vi "_Validate Source Parameters.vi"(11 "Expts":string[][](array[string])=[["0", "MRM", "Positive", "234", "7199", "22", "5000", "20", "2", "70", "ESI1 5001"], ["1", "MRM", "Positive", "0", "4988", "22", "5000", "0", "2", "70", "APCI2 3.1"], ["2", "MRM", "Negative", "678", "9085", "22", "5000", "20", "2", "70", "ESI1 -4001"], ["3", "MRM", "Negative", "0", "7199", "22", "5000", "0", "2", "70", "APCI2 -3.2"]]) -> (1 "Error":string, 2 "SourceProperties":T2[](array[typedef])=[{"Source Type"=2, "IsPole1"=TRUE, "IsAPCI"=FALSE, "IsPositive"=TRUE, "CD"=0.0, "ES1"=5001.0, "ES2"=0.0, "NextCD"=0.0, "NextES1"=0.0, "NextES2"=0.0, "PolSwitching"=FALSE, "StartTime"=0.0, "StopTime"=7199.0, "DelayTime"=20.0, "Cycles"=0, "PauseTime"=0.0, "ExptDuration"=0.0}, {"Source Type"=1, "IsPole1"=FALSE, "IsAPCI"=TRUE, "IsPositive"=TRUE, "CD"=3.1, "ES1"=0.0, "ES2"=0.0, "NextCD"=0.0, "NextES1"=0.0, "NextES2"=0.0, "PolSwitching"=FALSE, "StartTime"=0.0, "StopTime"=7199.0, "DelayTime"=0.0, "Cycles"=0, "PauseTime"=0.0, "ExptDuration"=0.0}, {"Source Type"=2, "IsPole1"=TRUE, "IsAPCI"=FALSE, "IsPositive"=FALSE, "CD"=0.0, "ES1"=-4001.0, "ES2"=0.0, "NextCD"=0.0, "NextES1"=0.0, "NextES2"=0.0, "PolSwitching"=FALSE, "StartTime"=0.0, "StopTime"=7199.0, "DelayTime"=20.0, "Cycles"=0, "PauseTime"=0.0, "ExptDuration"=0.0}, {"Source Type"=1, "IsPole1"=FALSE, "IsAPCI"=TRUE, "IsPositive"=FALSE, "CD"=-3.2, "ES1"=0.0, "ES2"=0.0, "NextCD"=0.0, "NextES1"=0.0, "NextES2"=0.0, "PolSwitching"=FALSE, "StartTime"=0.0, "StopTime"=7199.0, "DelayTime"=0.0, "Cycles"=0, "PauseTime"=0.0, "ExptDuration"=0.0}] {"Source Type" items=["APCI 1", "APCI 2", "ESI 1", "ESI 2"]}, 3 "Valid":bool)   [LabVIEW 2012]
uses:
  _Source Properties.ctl
  _XML Source Type.ctl
panel:
  out "PeriodList":T1(array[cluster])
  out "Time array":dbl[](array[numeric])
  # "Num             Type            Polarity        StartTime      StopTime        Cycles       PauseTime    DelayTime      ExptDur      DwellTime   Comment"
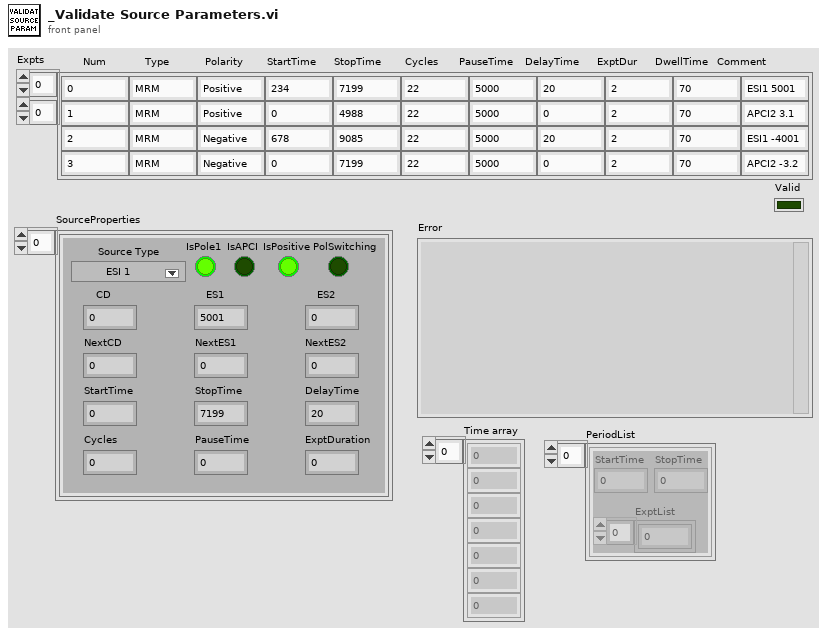
[diagram p1: front panel]
types:
  T1 = cluster{"StartTime":dbl, "StopTime":dbl, "ExptList":i32[]}[]
  T2 = typedef "_Source Properties.ctl" = cluster{"Source Type":T3, "IsPole1":bool, "IsAPCI":bool, "IsPositive":bool, "CD":dbl, "ES1":dbl, "ES2":dbl, "NextCD":dbl, "NextES1":dbl, "NextES2":dbl, "PolSwitching":bool, "StartTime":dbl, "StopTime":dbl, "DelayTime":dbl, "Cycles":i32, "PauseTime":dbl, "ExptDuration":dbl}
  T3 = typedef "_XML Source Type.ctl" = u16
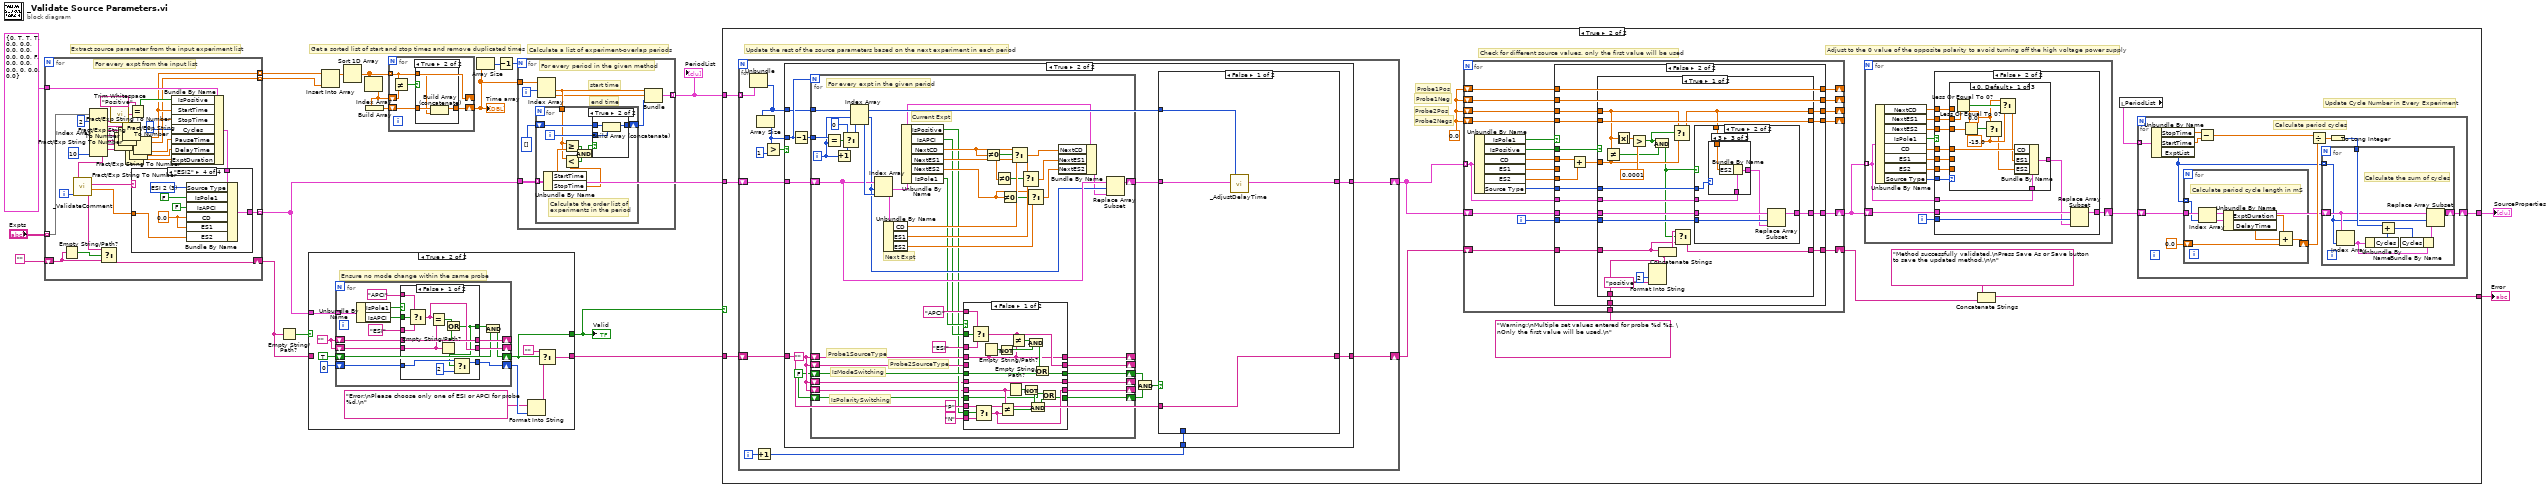
[diagram p0: block diagram]
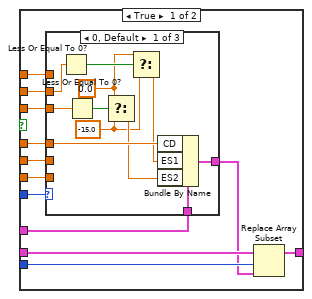
[diagram p3: hidden frame]
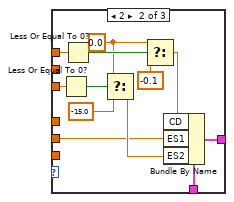
[diagram p4: hidden frame]
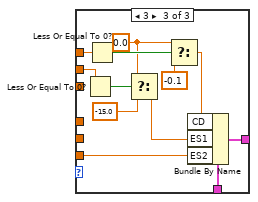
[diagram p5: hidden frame]
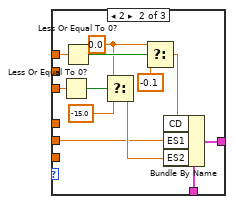
[diagram p6: hidden frame]
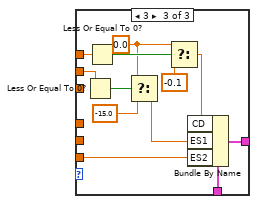
[diagram p7: hidden frame]
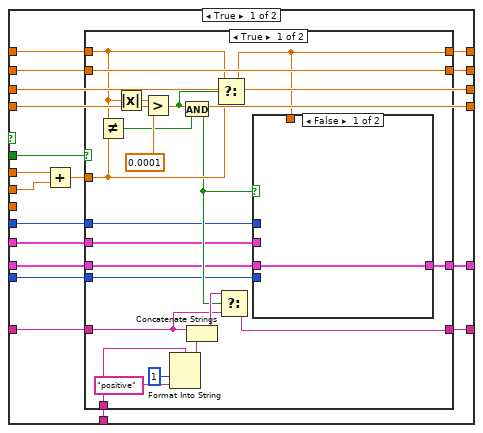
[diagram p8: hidden frame]
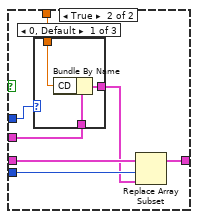
[diagram p9: hidden frame]
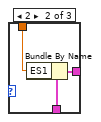
[diagram p10: hidden frame]
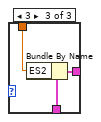
[diagram p11: hidden frame]
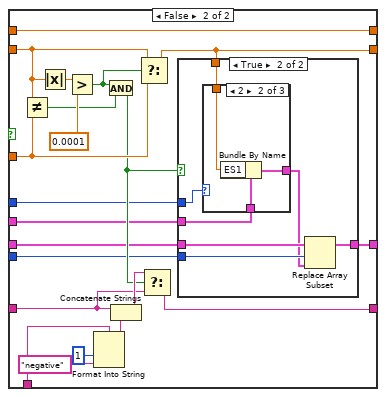
[diagram p12: hidden frame]
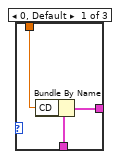
[diagram p14: hidden frame]
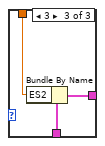
[diagram p15: hidden frame]
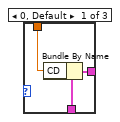
[diagram p17: hidden frame]
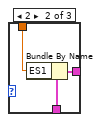
[diagram p18: hidden frame]
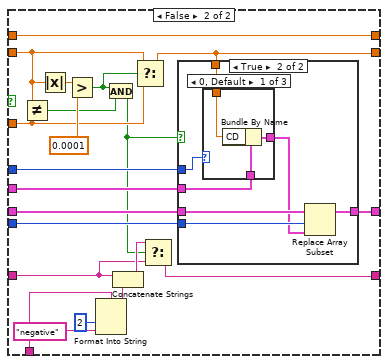
[diagram p19: hidden frame]
diagram:
  # "Extract source parameter from the input experiment list"
  # "Calculate a list of experiment-overlap periods"
  # "Get a sorted list of start and stop times and remove duplicated times"
  n1 = for {
    tunnel: "Expts" -> [w50] mode=indexing
    tunnel: T2 {"Source Type"=0, "IsPole1"=TRUE, "IsAPCI"=TRUE, "IsPositive"=TRUE, "CD"=0.0, "ES1"=0.0, "ES2"=0.0, "NextCD"=0.0, "NextES1"=0.0, "NextES2"=0.0, "PolSwitching"=FALSE, "StartTime"=0.0, "StopTime"=0.0, "DelayTime"=0.0, "Cycles"=0, "PauseTime"=0.0, "ExptDuration"=0.0} ("SourceParameters") -> [w42]
    tunnel: [w39] -> w8 mode=indexing
    tunnel: [w38] -> w18 mode=indexing
    tunnel: [w37] -> w17 mode=indexing
    shift-right: [w30] -> w3
    shift-left: "" -> [w31]
    i -> [w36]
    # "For every expt from the input list"
    n2 = Empty String/Path?(string/path=w31) -> (empty?=w33:bool)
    n3 = Index Array(array=w50, index #1=2 ("index"), index #8=10 ("index")) -> (element #1=w48:string, element #2=w43:string, element #3=w44:string, element #4=w45:string, element #5=w29:string, element #6=w28:string, element #7=w27:string, element #8=w23:string)  [unwired: 6 in]
    n4 = call "_ValidateComment.vi"("Expt#"=w36, "Comment"=w23) -> ("Error"=w32:string, "ParamValue"=w34:dbl, "SourceType"=w35:string)  [unwired: 2 in, 1 out]
    n5 = Select(t=w32, s=w33, f=w31) -> (s? t:f=w30:string)
    n6 = call <vilib>:"Trim Whitespace.vi"("string"=w48) -> ("trimmed string"=w47:string)  [unwired: 1 in]
    n7 = Fract/Exp String To Number(string=w45) -> ()  [unwired: 3 in, 2 out]
    n8 = Fract/Exp String To Number(string=w44) -> (number=w37:dbl)  [unwired: 3 in, 1 out]
    n9 = Fract/Exp String To Number(string=w43) -> (number=w38:dbl)  [unwired: 3 in, 1 out]
    n10 = Fract/Exp String To Number(string=w27) -> (number=w22:dbl)  [unwired: 3 in, 1 out]
    n11 = Equal?(x="Positive", y=w47) -> (x = y?=w41:bool)
    n12 = Fract/Exp String To Number(string=w28) -> (number=w25:dbl)  [unwired: 3 in, 1 out]
    n13 = Fract/Exp String To Number(string=w29) -> (number=w26:dbl)  [unwired: 3 in, 1 out]
    n14 = Bundle By Name(cluster=w42, "IsPositive"=w41, "StartTime"=w38, "StopTime"=w37, "Cycles"=0, "PauseTime"=w26, "DelayTime"=w25, "ExptDuration"=w22) -> (w40:T2)
    n15 = case shown="\"ESI2\"" w35 {
      tunnel: w40 -> [w56 w63 w70 w77]
      tunnel: w34 -> [w53 w60 w65 w72]
      tunnel: [w51 w57 w64 w71] -> w39
      frame "APCI1", Default {
        w52 = 0.0 ("ES1")
        w54 = TRUE ("IsPole1")
        w55 = T3 0 items=["APCI 1", "APCI 2", "ESI 1", "ESI 2"] ("Source Type")
        n16 = Bundle By Name(cluster=w56, "Source Type"=w55, "IsPole1"=w54, "IsAPCI"=w54, "CD"=w53, "ES1"=w52, "ES2"=w52) -> (w51:T2)
      }
      frame "APCI2" {
        w59 = 0.0 ("ES1")
        w62 = T3 1 items=["APCI 1", "APCI 2", "ESI 1", "ESI 2"] ("Source Type")
        n17 = Bundle By Name(cluster=w63, "Source Type"=w62, "IsPole1"=FALSE, "IsAPCI"=TRUE, "CD"=w60, "ES1"=w59, "ES2"=w59) -> (w57:T2)
      }
      frame "ESI1" {
        w66 = 0.0 ("ES1")
        w69 = T3 2 items=["APCI 1", "APCI 2", "ESI 1", "ESI 2"] ("Source Type")
        n18 = Bundle By Name(cluster=w70, "Source Type"=w69, "IsPole1"=TRUE, "IsAPCI"=FALSE, "CD"=w66, "ES1"=w65, "ES2"=w66) -> (w64:T2)
      }
      frame "ESI2" {
        w73 = 0.0 ("ES1")
        w76 = T3 3 items=["APCI 1", "APCI 2", "ESI 1", "ESI 2"] ("Source Type")
        n19 = Bundle By Name(cluster=w77, "Source Type"=w76, "IsPole1"=FALSE, "IsAPCI"=FALSE, "CD"=w73, "ES1"=w73, "ES2"=w72) -> (w71:T2)
      }
    }
  }
  n20 = Empty String/Path?(string/path=w3) -> (empty?=w4:bool)
  n21 = case shown="True" w4 {
    selector: w4 -> [w79 _]
    tunnel: w8 -> [_ w82]
    tunnel: [w78 w81] -> w7
    tunnel: [w79 w80] -> w1
    tunnel: w3 -> [w78 _]
    frame False {
    }
    frame True {
      w89 = ""
      # "Ensure no mode change within the same probe"
      n22 = for {
        tunnel: w82 -> [w103] mode=indexing
        shift-right: [w98] -> _
        shift-left: w89 -> [w101]
        shift-right: [w99] -> _
        shift-left: w89 -> [w100]
        shift-right: [w92] -> w80
        shift-left: TRUE -> [w93]
        shift-right: [w90] -> w85
        shift-left: 0 -> [w91]
        n23 = Unbundle By Name(w103) -> ("IsPole1"=w102:bool, "IsAPCI"=w97:bool)
        n24 = case shown="False" w102 {
          tunnel: w101 -> [w115 w123]
          tunnel: w100 -> [w110 w127]
          tunnel: [w109 w127] -> w99
          tunnel: [w115 w120] -> w98
          tunnel: w97 -> [w113 w126]
          tunnel: "APCI" -> [w112 w125]
          tunnel: "ESI" -> [w111 w124]
          tunnel: [w106 w119] -> w94
          tunnel: [w104 w116] -> w90
          tunnel: w91 -> [w107 w118]
          frame False {
            n25 = Select(t=w112, s=w113, f=w111) -> (s? t:f=w109:string)
            n26 = Equal?(x=w109, y=w110) -> (x = y?=w114:bool)
            n27 = Empty String/Path?(string/path=w110) -> (empty?=w108:bool)
            n28 = Or(x=w114, y=w108) -> (x .or. y?=w106:bool)
            n29 = Select(t=w107, s=w106, f=2) -> (s? t:f=w104:i32)
          }
          frame True {
            n30 = Select(t=w125, s=w126, f=w124) -> (s? t:f=w120:string)
            n31 = Equal?(x=w120, y=w123) -> (x = y?=w121:bool)
            n32 = Empty String/Path?(string/path=w123) -> (empty?=w122:bool)
            n33 = Or(x=w121, y=w122) -> (x .or. y?=w119:bool)
            n34 = Select(t=w118, s=w119, f=1) -> (s? t:f=w116:i32)
          }
        }
        n35 = And(x=w94, y=w93) -> (x .and. y?=w92:bool)
      }
      n36 = Format Into String(format string="Error:\nPlease choose only one of ESI or APCI for probe %d.\n", w85) -> (resulting string=w83:string)  [unwired: 2 in, 1 out]
      n37 = Select(t="", s=w80, f=w83) -> (s? t:f=w81:string)
    }
  }
  "Valid" <- w1
  n38 = Insert Into Array(array=w18, new element=w17) -> (w16:dbl[])  [unwired: 1 in]
  n39 = Sort 1D Array(array=w16) -> (sorted array=w15:dbl[])
  n40 = Index Array(array=w15) -> (element=w14:dbl)  [unwired: 1 in]
  n41 = Build Array(w14) -> (w13:dbl[])
  n42 = for {
    tunnel: w15 -> [w128] mode=indexing
    shift-right: [w128] -> _
    shift-left: w14 -> [w132]
    shift-right: [w129] -> w10
    shift-left: w13 -> [w130]
    n43 = Not Equal?(x=w128, y=w132) -> (x != y?=w131:bool)
    n44 = case shown="True" w131 {
      tunnel: w128 -> [_ w134]
      tunnel: w130 -> [w133 w136]
      tunnel: [w133 w135] -> w129
      frame False {
      }
      frame True {
        n45 = Build Array (concatenate)(w136, w134) -> (w135:dbl[])
      }
    }
  }
  "Time array" <- w10
  n46 = Array Size(array=w10) -> (size(s)=w12:i32)
  n47 = Decrement(x=w12) -> (x-1=w11:i32)
  n48 = for {
    N: w11 -> [_]
    tunnel: w8 -> [w142]
    tunnel: w10 -> [w144]
    tunnel: [w137] -> w9 mode=indexing
    i -> [w143]
    # "For every period in the given method"
    # "end time"
    # "start time"
    n49 = Index Array(array=w144, index #1=w143) -> (element #1=w140:dbl, element #2=w139:dbl)  [unwired: 1 in]
    n50 = for {
      tunnel: w142 -> [w154] mode=indexing
      tunnel: w140 -> [w148]
      shift-right: [w150] -> w138
      shift-left: i32[] [] ("output array") -> [w151]
      i -> [w152]
      # "Calculate the order list of\nexperiments in the period"
      n51 = Unbundle By Name(w154) -> ("StartTime"=w153:dbl, "StopTime"=w149:dbl)
      n52 = Greater Or Equal?(x=w148, y=w153) -> (x >= y?=w147:bool)
      n53 = Less?(x=w148, y=w149) -> (x < y?=w146:bool)
      n54 = And(x=w147, y=w146) -> (x .and. y?=w145:bool)
      n55 = case shown="True" w145 {
        tunnel: w152 -> [_ w157]
        tunnel: w151 -> [w155 w158]
        tunnel: [w155 w156] -> w150
        frame False {
        }
        frame True {
          n56 = Build Array (concatenate)(w158, w157) -> (w156:i32[])
        }
      }
    }
    n57 = Bundle(w140, w139, "output array"=w138) -> (w137:cluster{dbl, dbl, "output array":i32[]})  [unwired: 1 in]
  }
  "PeriodList" <- w9
  n58 = case shown="True" w1 {
    tunnel: w9 -> [_ w173]
    tunnel: w8 -> [_ w172]
    tunnel: w7 -> [w159 w171]
    tunnel: [_ w161] -> w6
    tunnel: [w159 w165] -> w2
    frame False {
    }
    frame True {
      w169 = 0.0
      # "Update Cycle Number in Every Experiment"
      # "Adjust to the 0 value of the opposite polarity to avoid turning off the high voltage power supply"
      # "Probe2Negs"
      # "Probe2Pos"
      # "Probe1Neg"
      # "Probe1Pos"
      # "Check for different source values, only the first value will be used"
      # "Update the rest of the source parameters based on the next experiment in each period"
      n59 = for {
        tunnel: w173 -> [w516] mode=indexing
        shift-right: [w522] -> w167
        shift-left: w172 -> [w523]
        shift-right: [w517] -> w170
        shift-left: w171 -> [w518]
        i -> [w520]
        n60 = Unbundle(w516) -> ("output array"=w515:i32[])  [unwired: 2 out]
        n61 = Increment(x=w520) -> (x+1=w519:i32)
        n62 = Array Size(array=w515) -> (size(s)=w521:i32)
        n63 = Greater?(x=w521, y=1) -> (0:w524:bool)
        n64 = case shown="True" w524 {
          tunnel: w523 -> [w527 w541]
          tunnel: [w527 w534] -> w522
          tunnel: w515 -> [_ w532]
          tunnel: w521 -> [_ w533]
          tunnel: w519 -> [_ w530]
          tunnel: [w526 w529] -> w517
          tunnel: w518 -> [w526 w528]
          frame False {
            # "No experiment overlap in this period"
          }
          frame True {
            w539 = FALSE
            w540 = ""
            n65 = Decrement(x=w533) -> (x-1=w531:i32)
            n66 = for {
              N: w533 -> [_]
              tunnel: w532 -> [w595]
              tunnel: w531 -> [w599]
              shift-right: [w586] -> w535
              shift-left: w541 -> [w589]
              shift-right: [w569] -> _
              shift-left: w540 -> [w568]
              shift-right: [w567] -> _
              shift-left: w540 -> [w566]
              shift-right: [w564] -> w538
              shift-left: w539 -> [w565]
              shift-right: [w560] -> _
              shift-left: w540 -> [w559]
              shift-right: [w558] -> _
              shift-left: w540 -> [w557]
              shift-right: [w555] -> w537
              shift-left: w539 -> [w556]
              i -> [w594]
              # "IsPolaritySwitching"
              # "Probe2SourceType"
              # "Probe1SourceType"
              # "IsModeSwitching"
              # "For every expt in the given period"
              # "Next Expt"
              # "Current Expt"
              n67 = Equal?(x=w599, y=w594) -> (x = y?=w598:bool)
              n68 = Increment(x=w594) -> (x+1=w597:i32)
              n69 = Select(t=0, s=w598, f=w597) -> (s? t:f=w593:i32)
              n70 = Index Array(array=w595, index #1=w594, index #2=w593) -> (element #1=w588:i32, element #2=w592:i32)
              n71 = Index Array(array=w589, index #1=w588, index #2=w592) -> (element #1=w590:T2, element #2=w591:T2)
              n72 = Unbundle By Name(w591) -> ("CD"=w583:dbl, "ES1"=w579:dbl, "ES2"=w576:dbl)
              n73 = Unbundle By Name(w590) -> ("IsPositive"=w561:bool, "IsAPCI"=w570:bool, "NextCD"=w585:dbl, "NextES1"=w580:dbl, "NextES2"=w574:dbl, "IsPole1"=w571:bool)
              n74 = case shown="False" w571 {
                tunnel: w568 -> [w612 _]
                tunnel: w566 -> [_ w641]
                tunnel: [w613 w641] -> w567
                tunnel: [w612 w642] -> w569
                tunnel: w570 -> [w622 w645]
                tunnel: "APCI" -> [w621 w644]
                tunnel: "ESI" -> [w620 w643]
                tunnel: w565 -> [w615 w636]
                tunnel: [w614 w635] -> w564
                tunnel: "P" -> [w611 w628]
                tunnel: "N" -> [w610 w627]
                tunnel: w561 -> [w609 w629]
                tunnel: [w608 w624] -> w560
                tunnel: w559 -> [w608 w626]
                tunnel: [w607 w634] -> w558
                tunnel: w557 -> [w605 w634]
                tunnel: w556 -> [w601 w625]
                tunnel: [w600 w623] -> w555
                frame False {
                  n75 = Select(t=w621, s=w622, f=w620) -> (s? t:f=w613:string)
                  n76 = Select(t=w611, s=w609, f=w610) -> (s? t:f=w607:string)
                  n77 = Empty String/Path?(string/path=w612) -> (empty?=w618:bool)
                  n78 = Not(x=w618) -> (.not. x?=w617:bool)
                  n79 = Not Equal?(x=w605, y=w607) -> (x != y?=w603:bool)
                  n80 = Empty String/Path?(string/path=w605) -> (empty?=w606:bool)
                  n81 = Not Equal?(x=w613, y=w612) -> (x != y?=w619:bool)
                  n82 = Not(x=w606) -> (.not. x?=w604:bool)
                  n83 = And(x=w619, y=w617) -> (x .and. y?=w616:bool)
                  n84 = And(x=w604, y=w603) -> (x .and. y?=w602:bool)
                  n85 = Or(x=w616, y=w615) -> (x .or. y?=w614:bool)
                  n86 = Or(x=w601, y=w602) -> (x .or. y?=w600:bool)
                }
                frame True {
                  n87 = Select(t=w644, s=w645, f=w643) -> (s? t:f=w642:string)
                  n88 = Select(t=w628, s=w629, f=w627) -> (s? t:f=w624:string)
                  n89 = Empty String/Path?(string/path=w641) -> (empty?=w639:bool)
                  n90 = Not(x=w639) -> (.not. x?=w638:bool)
                  n91 = Not Equal?(x=w626, y=w624) -> (x != y?=w631:bool)
                  n92 = Not Equal?(x=w642, y=w641) -> (x != y?=w640:bool)
                  n93 = Empty String/Path?(string/path=w626) -> (empty?=w633:bool)
                  n94 = And(x=w640, y=w638) -> (x .and. y?=w637:bool)
                  n95 = Not(x=w633) -> (.not. x?=w632:bool)
                  n96 = Or(x=w637, y=w636) -> (x .or. y?=w635:bool)
                  n97 = And(x=w632, y=w631) -> (x .and. y?=w630:bool)
                  n98 = Or(x=w625, y=w630) -> (x .or. y?=w623:bool)
                }
              }
              n99 = Not Equal To 0?(x=w585) -> (x != 0?=w584:bool)
              n100 = Not Equal To 0?(x=w580) -> (x != 0?=w582:bool)
              n101 = Not Equal To 0?(x=w574) -> (x != 0?=w578:bool)
              n102 = Select(t=w585, s=w584, f=w583) -> (s? t:f=w581:dbl)
              n103 = Select(t=w580, s=w582, f=w579) -> (s? t:f=w577:dbl)
              n104 = Select(t=w574, s=w578, f=w576) -> (s? t:f=w575:dbl)
              n105 = Bundle By Name(cluster=w590, "NextCD"=w581, "NextES1"=w577, "NextES2"=w575) -> (w587:T2)
              n106 = Replace Array Subset(array=w589, new element=w587, index=w588) -> (w586:T2[])
            }
            n107 = And(x=w538, y=w537) -> (x .and. y?=w536:bool)
            n108 = case shown="False" w536 {
              selector: w536 -> [_ w546]
              tunnel: w535 -> [w544 w554]
              tunnel: [w543 w547] -> w534
              tunnel: w532 -> [w542 w553]
              tunnel: w530 -> [_ w551]
              tunnel: [w545 w548] -> w529
              tunnel: w528 -> [w545 w549]
              frame False {
                n109 = call "_AdjustDelayTime.vi"("SourceProperty in"=w544, "ExptList"=w542) -> ("SourceProperty out"=w543:T2[])  [unwired: 5 in]
              }
              frame True {
                # "for combined mode swithing and polarity switching segment, delay time of all experiments in the segment will be adjusted to at least 200mS"
                n110 = call "_AdjustDelayTime.vi"("CombinedModeAndPol"=w546, "SourceProperty in"=w554, "ExptList"=w553) -> ("SourceProperty out"=w547:T2[])  [unwired: 4 in]
                n111 = Format Into String(format string="Warning: \nSegment %d combines mode switching and polarity switching. \nData quality could be affected.\n", w551) -> (resulting string=w550:string)  [unwired: 2 in, 1 out]
                n112 = Concatenate Strings(w549, w550) -> (w548:string)
              }
            }
          }
        }
      }
      n113 = for {
        shift-right: [w315] -> w163
        shift-left: w170 -> [w316]
        shift-right: [w318] -> _
        shift-left: w169 -> [w324]
        shift-right: [w317] -> _
        shift-left: w169 -> [w323]
        shift-right: [w320] -> _
        shift-left: w169 -> [w322]
        shift-right: [w319] -> _
        shift-left: w169 -> [w321]
        tunnel: w167 -> [w312] mode=indexing
        tunnel: "Warning:\nMultiple set values entered for probe %d %s. \nOnly the first value will be used.\n" -> [w314]
        shift-right: [w310] -> w166
        shift-left: w167 -> [w311]
        i -> [w309]
        n114 = Unbundle By Name(w312) -> ("IsPole1"=w326:bool, "IsPositive"=w325:bool, "CD"=w308:dbl, "ES1"=w307:dbl, "ES2"=w306:dbl, "Source Type"=w313:T3)
        n115 = case shown="False" w326 {
          tunnel: w325 -> [w344 w438]
          tunnel: w324 -> [w343 w431]
          tunnel: w323 -> [w342 w430]
          tunnel: w322 -> [w341 w435]
          tunnel: w321 -> [w340 w434]
          tunnel: [w341 w432] -> w320
          tunnel: [w340 w433] -> w319
          tunnel: [w338 w431] -> w318
          tunnel: [w339 w430] -> w317
          tunnel: w316 -> [w337 w437]
          tunnel: [w336 w436] -> w315
          tunnel: w314 -> [w335 w429]
          tunnel: w313 -> [w334 w428]
          tunnel: w312 -> [w333 w427]
          tunnel: w311 -> [w332 w426]
          tunnel: [w331 w424] -> w310
          tunnel: w309 -> [w330 w425]
          tunnel: w308 -> [w328 w423]
          tunnel: w307 -> [w327 _]
          tunnel: w306 -> [_ w422]
          frame True {
            n116 = Add(x=w328, y=w327) -> (x+y=w329:dbl)
            n117 = case shown="True" w344 {
              tunnel: w343 -> [w360 w392]
              tunnel: w342 -> [w365 w391]
              tunnel: [w365 w383] -> w339
              tunnel: [w348 w392] -> w338
              tunnel: w329 -> [w359 w399]
              tunnel: w337 -> [w354 w394]
              tunnel: [w353 w393] -> w336
              tunnel: w335 -> [w352 w390]
              tunnel: w334 -> [w350 w388]
              tunnel: w333 -> [w349 w387]
              tunnel: w332 -> [w347 w386]
              tunnel: [w346 w384] -> w331
              tunnel: w330 -> [w345 w385]
              frame True {
                n118 = Not Equal?(x=w360, y=w359) -> (x != y?=w362:bool)
                n119 = Absolute Value(x=w360) -> (abs(x)=w364:dbl)
                n120 = Greater?(x=w364, y=0.0001) -> (0:w361:bool)
                n121 = Format Into String(format string=w352, 1 ("input 1"), "positive") -> (resulting string=w358:string)  [unwired: 2 in, 1 out]
                n122 = And(x=w361, y=w362) -> (x .and. y?=w351:bool)
                n123 = Concatenate Strings(w354, w358) -> (w355:string)
                n124 = Select(t=w360, s=w361, f=w359) -> (s? t:f=w348:dbl)
                n125 = Select(t=w355, s=w351, f=w354) -> (s? t:f=w353:string)
                n126 = case shown="False" w351 {
                  tunnel: w350 -> [_ w372]
                  tunnel: w349 -> [_ w373]
                  tunnel: w348 -> [_ w371]
                  tunnel: w347 -> [w366 w370]
                  tunnel: [w366 w368] -> w346
                  tunnel: w345 -> [_ w369]
                  frame False {
                  }
                  frame True {
                    n127 = case shown="0, Default" w372 {
                      tunnel: w373 -> [w376 w379 w382]
                      tunnel: w371 -> [w375 w378 w381]
                      tunnel: [w374 w377 w380] -> w367
                      frame 0, Default {
                        n128 = Bundle By Name(cluster=w376, "CD"=w375) -> (w374:T2)
                      }
                      frame 2 {
                        n129 = Bundle By Name(cluster=w379, "ES1"=w378) -> (w377:T2)
                      }
                      frame 3 {
                        n130 = Bundle By Name(cluster=w382, "ES2"=w381) -> (w380:T2)
                      }
                    }
                    n131 = Replace Array Subset(array=w370, new element=w367, index=w369) -> (w368:T2[])
                  }
                }
              }
              frame False {
                n132 = Not Equal?(x=w391, y=w399) -> (x != y?=w401:bool)
                n133 = Absolute Value(x=w391) -> (abs(x)=w403:dbl)
                n134 = Greater?(x=w403, y=0.0001) -> (0:w400:bool)
                n135 = Format Into String(format string=w390, 1 ("input 1"), "negative") -> (resulting string=w398:string)  [unwired: 2 in, 1 out]
                n136 = And(x=w400, y=w401) -> (x .and. y?=w389:bool)
                n137 = Concatenate Strings(w394, w398) -> (w395:string)
                n138 = Select(t=w391, s=w400, f=w399) -> (s? t:f=w383:dbl)
                n139 = Select(t=w395, s=w389, f=w394) -> (s? t:f=w393:string)
                n140 = case shown="True" w389 {
                  tunnel: w388 -> [_ w410]
                  tunnel: w387 -> [_ w411]
                  tunnel: w383 -> [_ w409]
                  tunnel: w386 -> [w404 w408]
                  tunnel: [w404 w406] -> w384
                  tunnel: w385 -> [_ w407]
                  frame False {
                  }
                  frame True {
                    n141 = case shown="2" w410 {
                      tunnel: w411 -> [w414 w417 w420]
                      tunnel: w409 -> [w413 w416 w419]
                      tunnel: [w412 w415 w418] -> w405
                      frame 0, Default {
                        n142 = Bundle By Name(cluster=w414, "CD"=w413) -> (w412:T2)
                      }
                      frame 2 {
                        n143 = Bundle By Name(cluster=w417, "ES1"=w416) -> (w415:T2)
                      }
                      frame 3 {
                        n144 = Bundle By Name(cluster=w420, "ES2"=w419) -> (w418:T2)
                      }
                    }
                    n145 = Replace Array Subset(array=w408, new element=w405, index=w407) -> (w406:T2[])
                  }
                }
              }
            }
          }
          frame False {
            n146 = Add(x=w423, y=w422) -> (x+y=w421:dbl)
            n147 = case shown="True" w438 {
              tunnel: w421 -> [w455 w493]
              tunnel: w437 -> [w450 w488]
              tunnel: [w449 w487] -> w436
              tunnel: w435 -> [w447 w486]
              tunnel: [w448 w478] -> w433
              tunnel: w434 -> [w448 w485]
              tunnel: [w440 w486] -> w432
              tunnel: w429 -> [w446 w484]
              tunnel: w428 -> [w445 w482]
              tunnel: w427 -> [w444 w483]
              tunnel: w426 -> [w443 w481]
              tunnel: w425 -> [w442 w480]
              tunnel: [w439 w477] -> w424
              frame True {
                n148 = Not Equal?(x=w447, y=w455) -> (x != y?=w457:bool)
                n149 = Absolute Value(x=w447) -> (abs(x)=w459:dbl)
                n150 = Greater?(x=w459, y=0.0001) -> (0:w456:bool)
                n151 = Format Into String(format string=w446, 2 ("input 1"), "positive") -> (resulting string=w454:string)  [unwired: 2 in, 1 out]
                n152 = And(x=w456, y=w457) -> (x .and. y?=w441:bool)
                n153 = Concatenate Strings(w450, w454) -> (w451:string)
                n154 = Select(t=w447, s=w456, f=w455) -> (s? t:f=w440:dbl)
                n155 = Select(t=w451, s=w441, f=w450) -> (s? t:f=w449:string)
                n156 = case shown="True" w441 {
                  tunnel: w445 -> [_ w466]
                  tunnel: w444 -> [_ w467]
                  tunnel: w440 -> [_ w465]
                  tunnel: w443 -> [w460 w464]
                  tunnel: [w460 w462] -> w439
                  tunnel: w442 -> [_ w463]
                  frame False {
                  }
                  frame True {
                    n157 = case shown="3" w466 {
                      tunnel: w467 -> [w470 w473 w476]
                      tunnel: w465 -> [w469 w472 w475]
                      tunnel: [w468 w471 w474] -> w461
                      frame 0, Default {
                        n158 = Bundle By Name(cluster=w470, "CD"=w469) -> (w468:T2)
                      }
                      frame 2 {
                        n159 = Bundle By Name(cluster=w473, "ES1"=w472) -> (w471:T2)
                      }
                      frame 3 {
                        n160 = Bundle By Name(cluster=w476, "ES2"=w475) -> (w474:T2)
                      }
                    }
                    n161 = Replace Array Subset(array=w464, new element=w461, index=w463) -> (w462:T2[])
                  }
                }
              }
              frame False {
                n162 = Not Equal?(x=w485, y=w493) -> (x != y?=w495:bool)
                n163 = Absolute Value(x=w485) -> (abs(x)=w497:dbl)
                n164 = Greater?(x=w497, y=0.0001) -> (0:w494:bool)
                n165 = Format Into String(format string=w484, 2 ("input 1"), "negative") -> (resulting string=w492:string)  [unwired: 2 in, 1 out]
                n166 = And(x=w494, y=w495) -> (x .and. y?=w479:bool)
                n167 = Concatenate Strings(w488, w492) -> (w489:string)
                n168 = Select(t=w485, s=w494, f=w493) -> (s? t:f=w478:dbl)
                n169 = Select(t=w489, s=w479, f=w488) -> (s? t:f=w487:string)
                n170 = case shown="True" w479 {
                  tunnel: w482 -> [_ w504]
                  tunnel: w483 -> [_ w505]
                  tunnel: w478 -> [_ w503]
                  tunnel: w481 -> [w498 w502]
                  tunnel: [w498 w500] -> w477
                  tunnel: w480 -> [_ w501]
                  frame False {
                  }
                  frame True {
                    n171 = case shown="0, Default" w504 {
                      tunnel: w505 -> [w508 w511 w514]
                      tunnel: w503 -> [w507 w510 w513]
                      tunnel: [w506 w509 w512] -> w499
                      frame 0, Default {
                        n172 = Bundle By Name(cluster=w508, "CD"=w507) -> (w506:T2)
                      }
                      frame 2 {
                        n173 = Bundle By Name(cluster=w511, "ES1"=w510) -> (w509:T2)
                      }
                      frame 3 {
                        n174 = Bundle By Name(cluster=w514, "ES2"=w513) -> (w512:T2)
                      }
                    }
                    n175 = Replace Array Subset(array=w502, new element=w499, index=w501) -> (w500:T2[])
                  }
                }
              }
            }
          }
        }
      }
      n176 = for {
        tunnel: w166 -> [w209] mode=indexing
        shift-right: [w207] -> w162
        shift-left: w166 -> [w208]
        i -> [w206]
        n177 = Unbundle By Name(w209) -> ("NextCD"=w202:dbl, "NextES1"=w201:dbl, "NextES2"=w200:dbl, "IsPole1"=w211:bool, "CD"=w205:dbl, "ES1"=w204:dbl, "ES2"=w203:dbl, "Source Type"=w210:T3)
        n178 = case shown="False" w211 {
          tunnel: w210 -> [w223 w270]
          tunnel: w209 -> [w222 w269]
          tunnel: w208 -> [w221 w268]
          tunnel: [w220 w267] -> w207
          tunnel: w206 -> [w219 w266]
          tunnel: w205 -> [w218 w265]
          tunnel: w204 -> [w215 w262]
          tunnel: w203 -> [w213 w260]
          tunnel: w202 -> [w214 w261]
          tunnel: w201 -> [w212 w259]
          tunnel: w200 -> [w217 w264]
          frame True {
            n179 = case shown="0, Default" w223 {
              tunnel: w222 -> [w234 w246 w258]
              tunnel: [w233 w245 w257] -> w216
              tunnel: w218 -> [w232 _ _]
              tunnel: w217 -> [w231 w244 _]
              tunnel: w215 -> [_ w240 _]
              tunnel: w214 -> [_ w238 w253]
              tunnel: w213 -> [_ _ w249]
              tunnel: w212 -> [w229 _ w248]
              frame 0, Default {
                w225 = -15.0 ("f")
                w226 = 0.0 ("t")
                n180 = Less Or Equal To 0?(x=w229) -> (x <= 0?=w227:bool)
                n181 = Less Or Equal To 0?(x=w231) -> (x <= 0?=w230:bool)
                n182 = Select(t=w226, s=w230, f=w225) -> (s? t:f=w228:dbl)
                n183 = Select(t=w226, s=w227, f=w225) -> (s? t:f=w224:dbl)
                n184 = Bundle By Name(cluster=w234, "CD"=w232, "ES1"=w224, "ES2"=w228) -> (w233:T2)
              }
              frame 2 {
                w237 = 0.0 ("t")
                n185 = Less Or Equal To 0?(x=w244) -> (x <= 0?=w243:bool)
                n186 = Less Or Equal To 0?(x=w238) -> (x <= 0?=w239:bool)
                n187 = Select(t=w237, s=w243, f=-15.0) -> (s? t:f=w241:dbl)
                n188 = Select(t=w237, s=w239, f=-0.1 ("ES1")) -> (s? t:f=w235:dbl)
                n189 = Bundle By Name(cluster=w246, "CD"=w235, "ES1"=w240, "ES2"=w241) -> (w245:T2)
              }
              frame 3 {
                w252 = 0.0 ("t")
                n190 = Less Or Equal To 0?(x=w248) -> (x <= 0?=w256:bool)
                n191 = Less Or Equal To 0?(x=w253) -> (x <= 0?=w254:bool)
                n192 = Select(t=w252, s=w256, f=-15.0) -> (s? t:f=w247:dbl)
                n193 = Select(t=w252, s=w254, f=-0.1 ("ES1")) -> (s? t:f=w250:dbl)
                n194 = Bundle By Name(cluster=w258, "CD"=w250, "ES1"=w247, "ES2"=w249) -> (w257:T2)
              }
            }
            n195 = Replace Array Subset(array=w221, new element=w216, index=w219) -> (w220:T2[])
          }
          frame False {
            n196 = case shown="0, Default" w270 {
              tunnel: w269 -> [w281 w293 w305]
              tunnel: [w280 w292 w304] -> w263
              tunnel: w265 -> [w279 _ _]
              tunnel: w264 -> [w278 w291 _]
              tunnel: w262 -> [_ w287 _]
              tunnel: w261 -> [_ w285 w300]
              tunnel: w260 -> [_ _ w296]
              tunnel: w259 -> [w275 _ w295]
              frame 0, Default {
                w273 = -15.0 ("f")
                w274 = 0.0 ("t")
                n197 = Less Or Equal To 0?(x=w275) -> (x <= 0?=w276:bool)
                n198 = Less Or Equal To 0?(x=w278) -> (x <= 0?=w277:bool)
                n199 = Select(t=w274, s=w277, f=w273) -> (s? t:f=w271:dbl)
                n200 = Select(t=w274, s=w276, f=w273) -> (s? t:f=w272:dbl)
                n201 = Bundle By Name(cluster=w281, "CD"=w279, "ES1"=w272, "ES2"=w271) -> (w280:T2)
              }
              frame 2 {
                w284 = 0.0 ("t")
                n202 = Less Or Equal To 0?(x=w291) -> (x <= 0?=w290:bool)
                n203 = Less Or Equal To 0?(x=w285) -> (x <= 0?=w286:bool)
                n204 = Select(t=w284, s=w290, f=-15.0) -> (s? t:f=w288:dbl)
                n205 = Select(t=w284, s=w286, f=-0.1 ("ES1")) -> (s? t:f=w282:dbl)
                n206 = Bundle By Name(cluster=w293, "CD"=w282, "ES1"=w287, "ES2"=w288) -> (w292:T2)
              }
              frame 3 {
                w299 = 0.0 ("t")
                n207 = Less Or Equal To 0?(x=w295) -> (x <= 0?=w303:bool)
                n208 = Less Or Equal To 0?(x=w300) -> (x <= 0?=w301:bool)
                n209 = Select(t=w299, s=w303, f=-15.0) -> (s? t:f=w294:dbl)
                n210 = Select(t=w299, s=w301, f=-0.1 ("ES1")) -> (s? t:f=w297:dbl)
                n211 = Bundle By Name(cluster=w305, "CD"=w297, "ES1"=w294, "ES2"=w296) -> (w304:T2)
              }
            }
            n212 = Replace Array Subset(array=w268, new element=w263, index=w266) -> (w267:T2[])
          }
        }
      }
      n213 = Concatenate Strings("Method successfully validated.\nPress Save As or Save button to save the updated method.\n\n", w163) -> (w165:string)
      n214 = local read "PeriodList"() -> (w160:T1)
      n215 = for {
        shift-right: [w176] -> w161
        shift-left: w162 -> [w177]
        tunnel: w160 -> [w174] mode=indexing
        # "Calculate period cycles"
        n216 = Unbundle By Name(w174) -> ("StopTime"=w184:dbl, "StartTime"=w183:dbl, "ExptList"=w178:i32[])
        n217 = for {
          tunnel: w178 -> [w198] mode=indexing
          tunnel: w177 -> [w199]
          shift-right: [w193] -> w180
          shift-left: 0.0 -> [w194]
          # "Calculate period cycle length in mS"
          n218 = Index Array(array=w199, index=w198) -> (element=w197:T2)
          n219 = Unbundle By Name(w197) -> ("ExptDuration"=w195:dbl, "DelayTime"=w196:dbl)
          n220 = Compound Arithmetic op=ADD(w195, w196, w194) -> (w193:dbl)
        }
        n221 = Subtract(x=w184, y=w183) -> (x-y=w181:dbl)
        n222 = Divide(x=w181, y=w180) -> (x/y=w179:dbl)
        n223 = To Long Integer(number=w179) -> (32bit integer=w175:i32)
        n224 = for {
          tunnel: w178 -> [w187] mode=indexing
          shift-right: [w185] -> w176
          shift-left: w177 -> [w188]
          tunnel: w175 -> [w191]
          # "Calculate the sum of cycles"
          n225 = Index Array(array=w188, index=w187) -> (element=w190:T2)
          n226 = Unbundle By Name(w190) -> ("Cycles"=w192:i32)
          n227 = Add(x=w191, y=w192) -> (x+y=w189:i32)
          n228 = Bundle By Name(cluster=w190, "Cycles"=w189) -> (w186:T2)
          n229 = Replace Array Subset(array=w188, new element=w186, index=w187) -> (w185:T2[])
        }
      }
    }
  }
  "SourceProperties" <- w6
  "Error" <- w2
